vi "SubTemplate_4x4x4_SetModifiedClassAttributes.vi"(6 "Unlock data if error? (T)":bool=TRUE, 8 "error in (no error)":errorcluster, 9 "Only unlock data? (F)":bool, 10 "Class attributes":T1, 11 "reference in":refnum<class "SubTemplate_4x4x4.lvclass">) -> (0 "error out":errorcluster, 3 "reference out":refnum<class "SubTemplate_4x4x4.lvclass">)   [LabVIEW 2020, in "SubTemplate_4x4x4.lvclass"]
doc: "This VI overwrites the class attributes associated with this class or subclass object reference and unlocks it for write access. If error in is set, the object is unlocked but its data will not be modified. If reference is wired, the class attributes of the class (or sub class) will be affected else the class attributes will default to this class.\n\nIn order to use this VI, you must first successfully lock the object's data using this class GetClassAttributesToModify VI."
uses:
  SubTemplate_4x4x4.lvclass
  protected/ClassAttributes.ctl
  BaseTemplate_4x4x4/protected/ClassAttributes.ctl
  SubTemplate_4x4x4.lvclass/SubTemplate_4x4x4.ctl
  vi.lib/addons/_goop3.llb/3GOOPStates.ctl
  BaseTemplate_4x4x4/BaseTemplate_4x4x4.lvclass
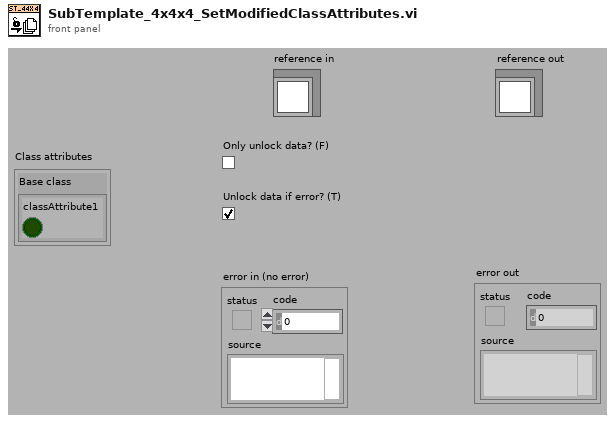
[diagram p1: front panel]
types:
  T1 = typedef "SubTemplate_4x4x4.lvclass/ClassAttributes.ctl" = cluster{"Base class":T2}
  T2 = typedef "BaseTemplate_4x4x4.lvclass/ClassAttributes.ctl" = cluster{"classAttribute1":bool}
  T3 = typedef "BaseTemplate_4x4x4.lvclass/ObjectReference.ctl" = refnum<k1>
  T4 = typedef "3GOOPStates.ctl" = enum16{"Set", "Get", "New", "Delete", "Clear", "Test and get", "Unlock data", "Information", "Look up existing", "New or look up existing", "Test and get shared", "Get shared", "Set shared", "Unlock shared", "Find dynamic method", "Register dynamic method", "Preload dynamic method", "Probe", "Cast to more generic", "Cast to more specific"}
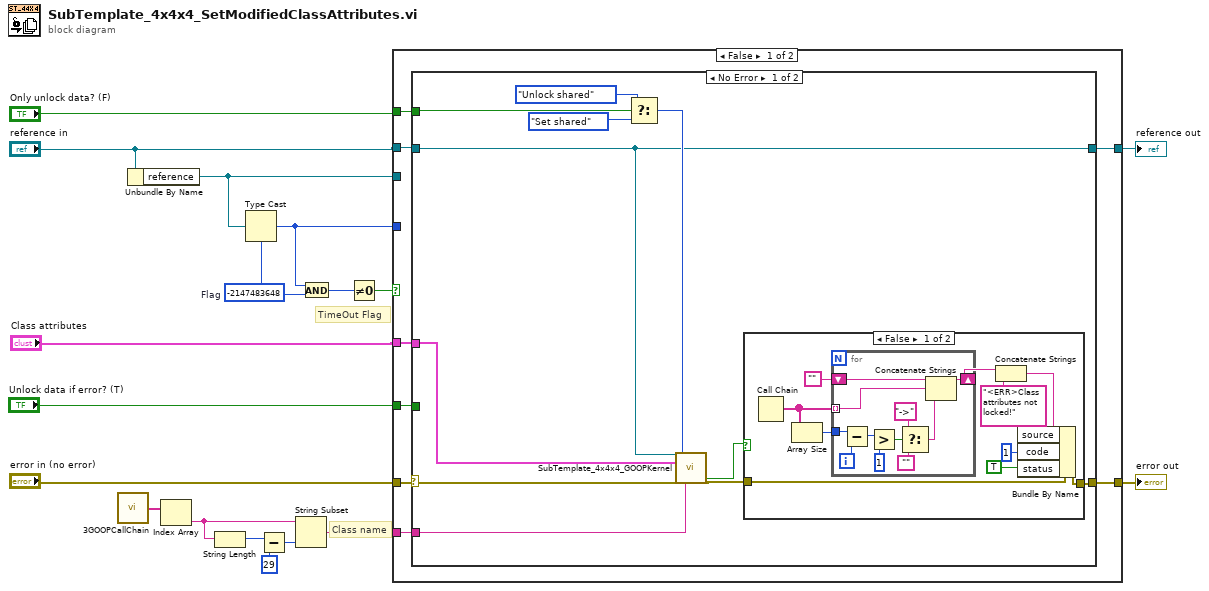
[diagram p0: block diagram]
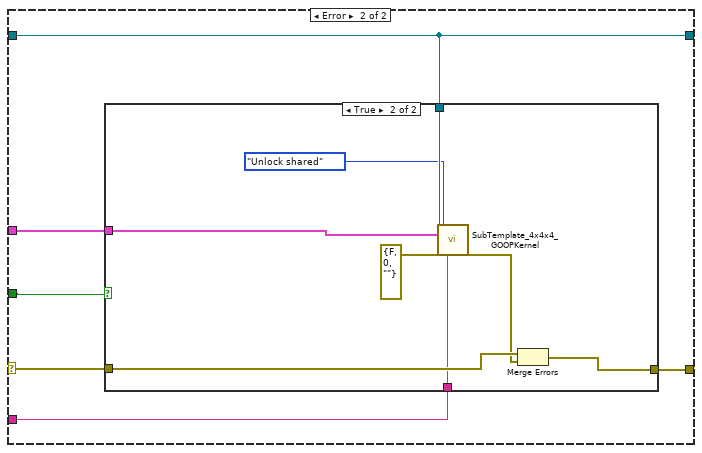
[diagram p3: hidden frame]
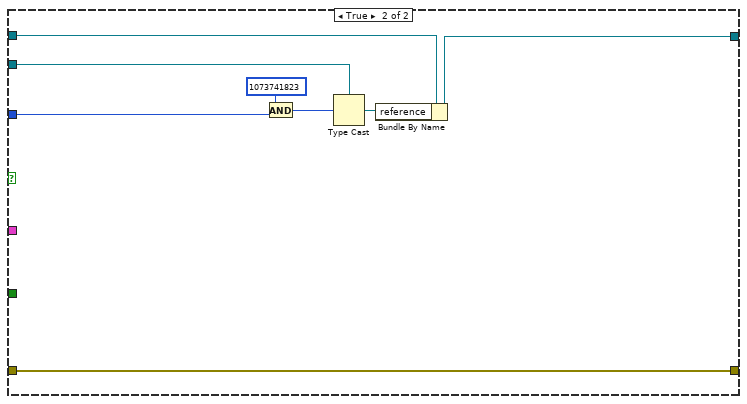
[diagram p5: hidden frame]
diagram:
  w10 = -2147483648  # Flag
  # "TimeOut Flag"
  # "Class name"
  n1 = call "3GOOPCallChain.vi"() -> ("call chain"=w15:string[])
  n2 = Unbundle By Name("reference in") -> ("reference"=w12:T3)
  n3 = Index Array(array=w15) -> (element=w18:string)  [unwired: 1 in]
  n4 = String Length(string=w18) -> (length=w14:i32)
  n5 = Type Cast(type=w10, x=w12) -> (*(type *) &x=w11:i32)
  n6 = Subtract(x=w14, y=29) -> (x-y=w16:i32)
  n7 = String Subset(string=w18, length (rest)=w16) -> (substring=w5:string)  [unwired: 1 in]
  n8 = And(x=w11, y=w10) -> (x .and. y?=w13:i32)
  n9 = Not Equal To 0?(x=w13) -> (x != 0?=w1:bool)
  n10 = case shown="False" w1 {
    tunnel: "Unlock data if error? (T)" -> [w26 _]
    tunnel: "error in (no error)" -> [w25 w75]
    tunnel: "Class attributes" -> [w24 _]
    tunnel: "Only unlock data? (F)" -> [w23 _]
    tunnel: [w22 w78] -> w3
    tunnel: [w21 w75] -> w2
    tunnel: "reference in" -> [w20 w79]
    tunnel: w12 -> [_ w77]
    tunnel: w11 -> [_ w76]
    tunnel: w5 -> [w19 _]
    frame False {
      n11 = case shown="No Error" w25 {
        selector: w25 -> [w36 w63]
        tunnel: [w29 w61] -> w22
        tunnel: w24 -> [w28 w65]
        tunnel: [w32 w62] -> w21
        tunnel: w20 -> [w29 w61]
        tunnel: w23 -> [w37 _]
        tunnel: w26 -> [_ w64]
        tunnel: w19 -> [w27 w60]
        frame No Error {
          n12 = Select(t=3GOOPStates."Unlock shared" ("Action"), s=w37, f=3GOOPStates."Set shared" ("Action")) -> (s? t:f=w33:T4)
          n13 = call "SubTemplate_4x4x4_GOOPKernel.vi"("Ref in"=w29, "Data shared in"=w28, "error in (no error)"=w36, "Action"=w33, "Class name"=w27) -> ("Data locked?"=w30:bool, "error out"=w31:errorcluster)  [unwired: 12 in, 9 out]
          n14 = case shown="False" w30 {
            tunnel: w31 -> [w42 w59]
            tunnel: [w43 w59] -> w32
            frame False {
              n15 = Call Chain() -> (call chain=w38:string[])
              n16 = Array Size(array=w38) -> (size(s)=w46:i32)
              n17 = for {
                shift-right: [w52] -> w45
                shift-left: "" -> [w54]
                tunnel: w38 -> [w53] mode=indexing
                tunnel: w46 -> [w58]
                i -> [w57]
                n18 = Subtract(x=w58, y=w57) -> (x-y=w56:i32)
                n19 = Greater?(x=w56, y=1) -> (0:w49:bool)
                n20 = Select(t="->", s=w49, f="") -> (s? t:f=w48:string)
                n21 = Concatenate Strings(w54, w53, w48) -> (w52:string)
              }
              n22 = Concatenate Strings(w45, "<ERR>Class attributes not locked!" ("Bundle Element")) -> (w41:string)
              n23 = Bundle By Name(cluster=w42, "source"=w41, "code"=1, "status"=TRUE) -> (w43:errorcluster)
            }
            frame True {
            }
          }
        }
        frame Error {
          n24 = case shown="True" w64 {
            tunnel: w63 -> [w66 w73]
            tunnel: [w66 w74] -> w62
            tunnel: w65 -> [_ w68]
            tunnel: w61 -> [_ w70]
            tunnel: w60 -> [_ w67]
            frame False {
            }
            frame True {
              n25 = call "SubTemplate_4x4x4_GOOPKernel.vi"("Ref in"=w70, "Data shared in"=w68, "error in (no error)"=errorcluster {"status"=FALSE, "code"=0, "source"=""}, "Action"=3GOOPStates."Unlock shared", "Class name"=w67) -> ("error out"=w71:errorcluster)  [unwired: 12 in, 10 out]
              n26 = Merge Errors(w73, w71) -> (w74:errorcluster)
            }
          }
        }
      }
    }
    frame True {
      n27 = And(x=1073741823 ("x .and. y?"), y=w76) -> (x .and. y?=w82:i32)
      n28 = Type Cast(type=w77, x=w82) -> (*(type *) &x=w81:T3)
      n29 = Bundle By Name(cluster=w79, "reference"=w81) -> (w78:refnum<class "SubTemplate_4x4x4.lvclass">)
    }
  }
  "error out" <- w2
  "reference out" <- w3
